vi "_PC_D999_Var2StrArr.vi"(1 "DAQ String":string) -> (0 "Output":string[][](array[string]))   [LabVIEW 2018]
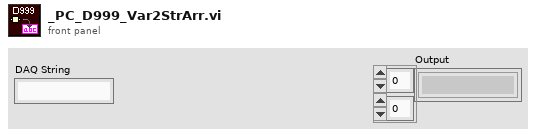
[diagram p1: front panel]
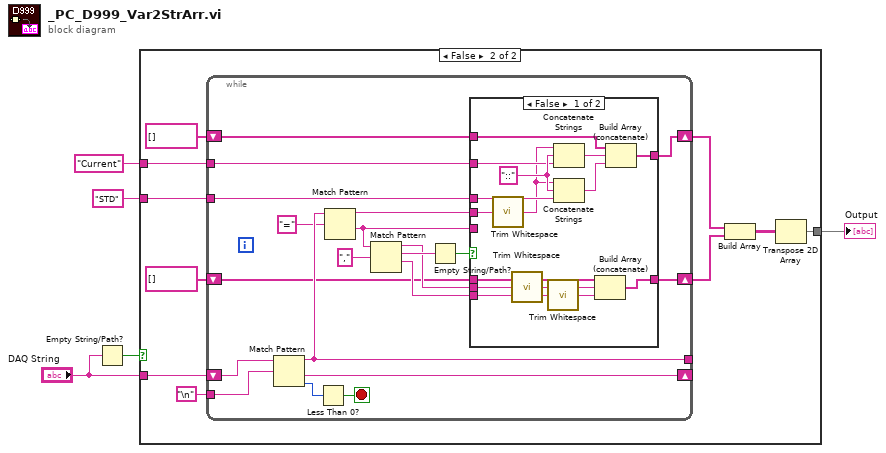
[diagram p0: block diagram]
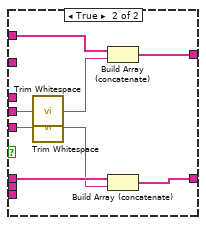
[diagram p3: hidden frame]
diagram:
  n1 = Empty String/Path?(string/path="DAQ String") -> (empty?=w2:bool)
  n2 = case shown="False" w2 {
    tunnel: "DAQ String" -> [_ w15]
    tunnel: [_ w13] -> w1
    tunnel: "Current" -> [_ w9]
    tunnel: "STD" -> [_ w8]
    frame True {
    }
    frame False {
      n3 = while {
        tunnel: "\n" -> [w34]
        tunnel: [w30] -> _
        shift-right: [w33] -> _
        shift-left: w15 -> [w32]
        shift-right: [w25] -> w12
        shift-left: string[] [] -> [w21]
        shift-right: [w24] -> w11
        shift-left: string[] [] -> [w20]
        tunnel: w9 -> [w19]
        tunnel: w8 -> [w18]
        stop <- w35 stop-if-true
        n4 = Match Pattern(string=w32, regular expression=w34) -> (before substring=w30:string, after substring=w33:string, offset past match=w31:i32)  [unwired: 1 in, 1 out]
        n5 = Less Than 0?(x=w31) -> (x < 0?=w35:bool)
        n6 = Match Pattern(string=w30, regular expression="=") -> (before substring=w17:string, after substring=w16:string)  [unwired: 1 in, 2 out]
        n7 = Match Pattern(string=w16, regular expression=",") -> (before substring=w23:string, match substring=w27:string, after substring=w22:string)  [unwired: 1 in, 1 out]
        n8 = Empty String/Path?(string/path=w27) -> (empty?=w26:bool)
        n9 = case shown="False" w26 {
          tunnel: [w47 w55] -> w25
          tunnel: w17 -> [w41 w57]
          tunnel: [w46 w52] -> w24
          tunnel: w16 -> [_ w58]
          tunnel: w23 -> [w39 _]
          tunnel: w22 -> [w37 _]
          tunnel: w21 -> [w45 w56]
          tunnel: w20 -> [w44 w53]
          tunnel: w19 -> [w43 _]
          tunnel: w18 -> [w42 _]
          frame False {
            w50 = "::"
            n10 = call <vilib>:"Trim Whitespace.vi"("string"=w41) -> ("trimmed string"=w40:string)  [unwired: 1 in]
            n11 = call <vilib>:"Trim Whitespace.vi"("string"=w39) -> ("trimmed string"=w38:string)  [unwired: 1 in]
            n12 = call <vilib>:"Trim Whitespace.vi"("string"=w37) -> ("trimmed string"=w36:string)  [unwired: 1 in]
            n13 = Concatenate Strings(w40, w50, w43) -> (w49:string)
            n14 = Concatenate Strings(w40, w50, w42) -> (w48:string)
            n15 = Build Array (concatenate)(w44, w38, w36) -> (w46:string[])
            n16 = Build Array (concatenate)(w45, w49, w48) -> (w47:string[])
          }
          frame True {
            n17 = call <vilib>:"Trim Whitespace.vi"("string"=w57) -> ("trimmed string"=w54:string)  [unwired: 1 in]
            n18 = call <vilib>:"Trim Whitespace.vi"("string"=w58) -> ("trimmed string"=w51:string)  [unwired: 1 in]
            n19 = Build Array (concatenate)(w56, w54) -> (w55:string[])
            n20 = Build Array (concatenate)(w53, w51) -> (w52:string[])
          }
        }
      }
      n21 = Build Array(w12, w11) -> (w10:string[][])
      n22 = Transpose 2D Array(2D array=w10) -> (transposed array=w13:string[][])
    }
  }
  "Output" <- w1
